vi "Prober_ChuckStatusCheck.vi"(8 "error in (no error)":errorcluster, 11 "TeslaVeloxProbeStation in":refnum<class "TeslaVeloxProbeStation.lvclass">) -> (0 "error out":errorcluster, 2 "Chuck at CONTACT?":bool=TRUE, 3 "TeslaVeloxProbeStation out":refnum<class "TeslaVeloxProbeStation.lvclass">)   [LabVIEW 2018, in "TeslaVeloxProbeStation.lvclass"]
uses:
  TeslaVeloxProbeStation.lvclass
  Desktop/Kvasnicka/test_labview_library/Integration_toolkit_library/CascadeProbestation.lvlib
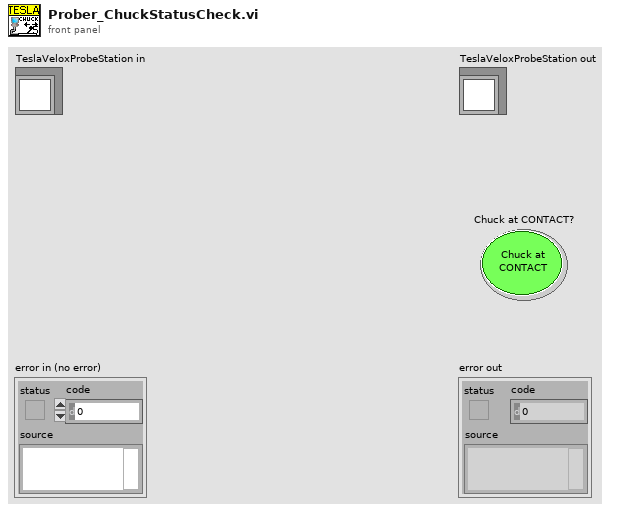
[diagram p1: front panel]
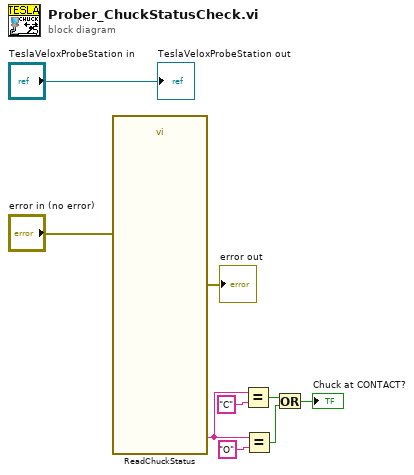
[diagram p0: block diagram]
diagram:
  n1 = call "ReadChuckStatus.vi"("Error In"="error in (no error)") -> ("Z Height"=w5:string, "Error Out"=→"error out":errorcluster)  [unwired: 7 in, 10 out]
  n2 = Equal?(x=w5, y="C") -> (x = y?=w4:bool)
  n3 = Equal?(x=w5, y="O") -> (x = y?=w3:bool)
  n4 = Or(x=w4, y=w3) -> (x .or. y?=→"Chuck at CONTACT?":bool)
  "TeslaVeloxProbeStation out" <- "TeslaVeloxProbeStation in"
